vi "Add Logging Section.vi"(8 "error in":errorcluster, 11 "custom device ref":T1 format="%.0x") -> (0 "error out":errorcluster, 1 "channel ref":T1 format="%.0x", 2 "logging":T1 format="%.0x", 3 "custom device ref out":T1 format="%.0x")   [LabVIEW 2020, in "AIM ARINC 664 Scripting.lvlib"]
uses:
  AIM ARINC 664 Scripting.lvlib
  <vilib>/NI VeriStand/Custom Device Offline API/Custom Device Offline API.lvlib
  Constants.vi
  <vilib>/NI VeriStand/Custom Device API/Custom Device API.lvlib
  <vilib>/NI VeriStand/Custom Device API/Custom Device Channel Type.ctl
  <vilib>/NI VeriStand/Custom Device API/Custom Device Channel.ctl
  <vilib>/NI VeriStand/Custom Device API/Custom Device Item Ref.ctl
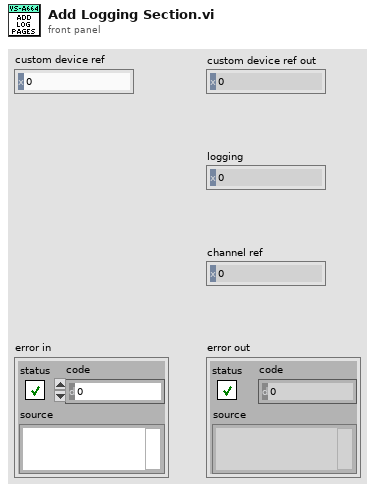
[diagram p1: front panel]
types:
  T1 = typedef "Custom Device API.lvlib/Custom Device Item Ref.ctl" = u64
  T2 = typedef "Custom Device API.lvlib/Custom Device Channel.ctl" = cluster{"Type":T3, "Units":string, "Default Value":dbl, "Faultable":bool, "Scalable":bool}
  T3 = typedef "Custom Device API.lvlib/Custom Device Channel Type.ctl" = enum16{"Input", "Output"}
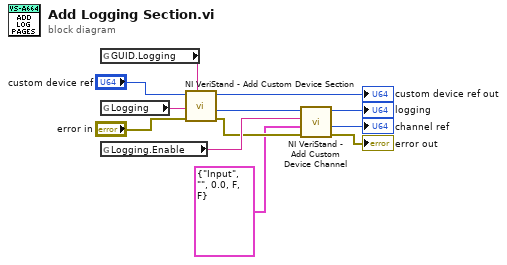
[diagram p0: block diagram]
diagram:
  n1 = global read "Constants.vi" "GUID.Logging"() -> (w8:string)
  n2 = global read "Constants.vi" "Logging"() -> (w9:string)
  n3 = global read "Constants.vi" "Logging.Enable"() -> (w5:string)
  n4 = call <vilib>:"NI VeriStand - Add Custom Device Section.vi"("GUID (Default Section)"=w8, "error in (no error)"="error in", "Section Name"=w9, "Parent Ref in"="custom device ref") -> ("error out"=w4:errorcluster, "Section Ptr"=w7:T1, "Parent Ref out"=→"custom device ref out":T1)  [unwired: 4 in, 1 out]
  n5 = call <vilib>:"NI VeriStand - Add Custom Device Channel.vi"("error in (no error)"=w4, "Channel"=T2 {"Type"=enum."Input", "Units"="", "Default Value"=0.0, "Faultable"=FALSE, "Scalable"=FALSE}, "Channel Name"=w5, "Parent Ref in"=w7) -> ("error out"=→"error out":errorcluster, "Channel Ref"=→"channel ref":T1, "Parent Ref out"=→"logging":T1)  [unwired: 4 in, 1 out]
